vi "Unregister for Waveform Data Events.vi"   [LabVIEW 2020, in "NI_VS Waveform Streaming Interface.lvlib"]
doc: "Unregisters all waveform data events associated with the event registration refnum. Event structures that use this event registration refnum no longer receive any events. Wire data to the <B>registered waveform data event (DBL)</B> input to determine the polymorphic instance to use or manually select the instance."
uses:
  <vilib>/NI VeriStand/Execution/WaveformStreaming/NI_VS Waveform Streaming Interface.lvlib
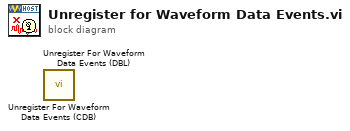
[diagram p0: block diagram]
diagram:
  n1 = call <vilib>:"Unregister For Waveform Data Events (CDB).vi"() -> ()  [unwired: 11 in, 1 out]
  n2 = call <vilib>:"Unregister For Waveform Data Events (DBL).vi"() -> ()  [unwired: 11 in, 1 out]
